vi "_FPGA Send Serial.vi"(4 "error in":errorcluster, 5 "Timeout (5000ms)":u32=5000, 6 "Serial Command":T1={"Port Type"=0, "baud rate (9600)"=9600, "data bits (8)"=8, "stop bits (1)"=10, "parity (0:none)"=0, "DoRead"=FALSE, "Command"=""} {"stop bits (1)" items=["1 bit"=10, "1.5 bits"=15, "2 bits"=20]; "parity (0:none)" items=["None", "Odd", "Even", "Mark", "Space"]; "data bits (8)" min=5 max=8 step=1; "Port Type" items=["RS485", "RS232-1", "RS232-2"]}) -> (0 "error out":errorcluster, 2 "Reply":string)   [LabVIEW 2015]
uses:
  Type/_RT Serial Command.ctl
  Type/_RW Status.ctl
  Type/_FPGA Indicator.ctl
  _RT Global.vi
  <vilib>/Utility/error.llb/Error Cluster From Error Code.vi
  <vilib>/rvi/errors/niLvFpgaAdjustHostInterfaceError.vi
  <vilib>/rvi/interface/nirviReadWriteControl/nirviReadWriteControl.xnode
  Type/FPGA Typedef.ctl
  FPGA Bitfiles/FPGA9607.lvbitx
  NiFpgaLv.dll
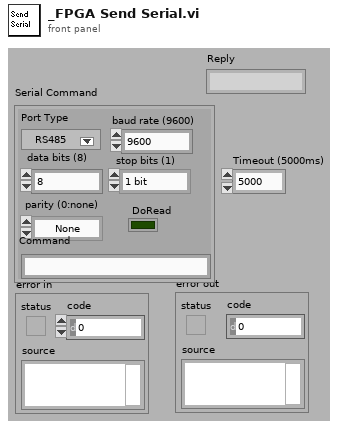
[diagram p1: front panel]
types:
  T1 = typedef "_RT Serial Command.ctl" = cluster{"Port Type":u16, "baud rate (9600)":u32, "data bits (8)":u16, "stop bits (1)":u16, "parity (0:none)":u16, "DoRead":bool, "Command":string}
  T2 = typedef "_RW Status.ctl" = enum8{"Done", "Do Read", "Do Write", "Set Latch1", "Set Latch2", "Set Latch3", "Set Latch4", "RP ON", "EL ON", "Serial Send", "Set LC Out", "Get LC In", "Read VAC", "Table Test", "Get Interlock", "Do Read2", "Do Write2"}
  T3 = typedef "FPGA Typedef.ctl" = refnum<k20>
  T4 = typedef "_FPGA Indicator.ctl" = enum16{"Done", "Ready", "Count Available", "SendSerial", "LED State"}
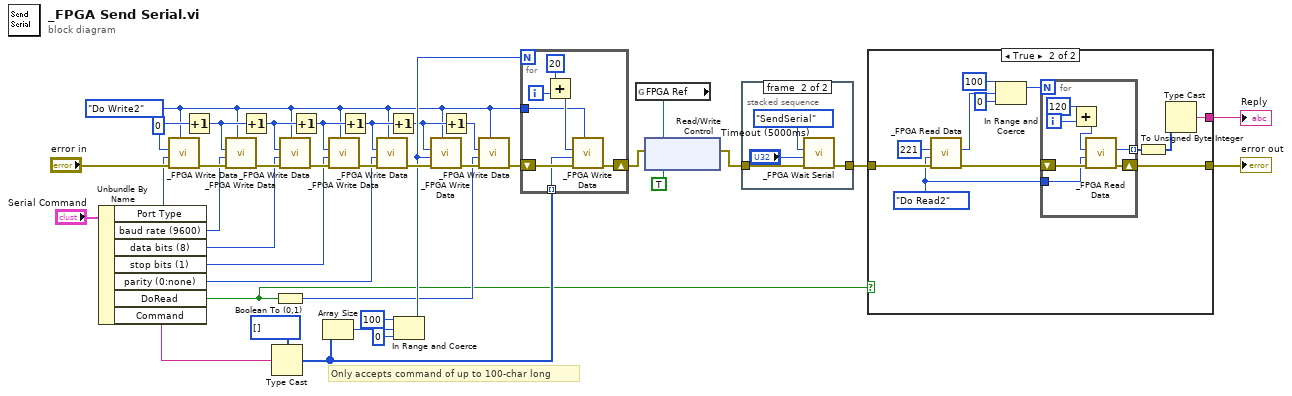
[diagram p0: block diagram]
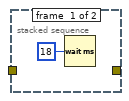
[diagram p3: hidden frame]
diagram:
  w4 = _RW_Status."Do Write2" ("Write Mode (Do Write)")
  w14 = u16 0 ("Address")
  # "Only accepts command of up to 100-char long"
  n1 = Unbundle By Name("Serial Command") -> ("Port Type"=w34:u16, "baud rate (9600)"=w33:u32, "data bits (8)"=w32:u16, "stop bits (1)"=w29:u16, "parity (0:none)"=w28:u16, "DoRead"=w2:bool, "Command"=w15:string)
  n2 = call "_FPGA Write Data.vi"("Write Mode (Do Write)"=w4, "error in"="error in", "Data"=w34, "Address"=w14) -> ("error out"=w37:errorcluster)  [unwired: 2 in, 2 out]
  n3 = Increment(x=w14) -> (x+1=w13:u16)
  n4 = call "_FPGA Write Data.vi"("Write Mode (Do Write)"=w4, "error in"=w37, "Data"=w33, "Address"=w13) -> ("error out"=w36:errorcluster)  [unwired: 2 in, 2 out]
  n5 = Increment(x=w13) -> (x+1=w12:u16)
  n6 = Type Cast(type=u8[] [], x=w15) -> (*(type *) &x=w21:u8[])
  n7 = Boolean To (0,1)(Boolean=w2) -> (0, 1=w8:i16)
  n8 = call "_FPGA Write Data.vi"("Write Mode (Do Write)"=w4, "error in"=w36, "Data"=w32, "Address"=w12) -> ("error out"=w30:errorcluster)  [unwired: 2 in, 2 out]
  n9 = Increment(x=w12) -> (x+1=w11:u16)
  n10 = Array Size(array=w21) -> (size(s)=w25:i32)
  n11 = call "_FPGA Write Data.vi"("Write Mode (Do Write)"=w4, "error in"=w30, "Data"=w29, "Address"=w11) -> ("error out"=w31:errorcluster)  [unwired: 2 in, 2 out]
  n12 = Increment(x=w11) -> (x+1=w10:u16)
  n13 = call "_FPGA Write Data.vi"("Write Mode (Do Write)"=w4, "error in"=w31, "Data"=w28, "Address"=w10) -> ("error out"=w26:errorcluster)  [unwired: 2 in, 2 out]
  n14 = Increment(x=w10) -> (x+1=w7:u16)
  n15 = In Range and Coerce(upper limit=100, x=w25, lower limit=0) -> (coerced(x)=w22:i32)  [unwired: 1 out]
  n16 = call "_FPGA Write Data.vi"("Write Mode (Do Write)"=w4, "error in"=w26, "Data"=w22, "Address"=w7) -> ("error out"=w9:errorcluster)  [unwired: 2 in, 2 out]
  n17 = Increment(x=w7) -> (x+1=w6:u16)
  n18 = call "_FPGA Write Data.vi"("Write Mode (Do Write)"=w4, "error in"=w9, "Data"=w8, "Address"=w6) -> ("error out"=w5:errorcluster)  [unwired: 2 in, 2 out]
  n19 = for {
    N: w22 -> [_]
    shift-right: [w42] -> w3
    shift-left: w5 -> [w43]
    tunnel: w21 -> [w40] mode=indexing
    tunnel: w4 -> [w39]
    i -> [w45]
    n20 = Add(x=20, y=w45) -> (x+y=w41:i32)
    n21 = call "_FPGA Write Data.vi"("Write Mode (Do Write)"=w39, "error in"=w43, "Data"=w40, "Address"=w41) -> ("error out"=w42:errorcluster)  [unwired: 2 in, 2 out]
  }
  n22 = global read "_RT Global.vi" "FPGA Ref"() -> (w1:T3)
  n23 = xnode "Read/Write Control"("FPGA VI Reference In"=w1, "error in"=w3, "Send Serial"=TRUE ("Start")) -> ("error out"=w19:errorcluster)  [unwired: 1 out]
  n24 = stacked-sequence {
    tunnel: w19 -> [_ w49]
    tunnel: [_ w48] -> w18
    frame #0 {
      n25 = Wait (ms)(milliseconds to wait=u32 18) -> ()  [unwired: 1 out]
    }
    frame #1 {
      n26 = call "_FPGA Wait Serial.vi"("error in"=w49, "Timeout (2000ms)"="Timeout (5000ms)", "Indicator"=_FPGA_Indicator."SendSerial") -> ("error out"=w48:errorcluster)  [unwired: 2 in, 2 out]
    }
  }
  n27 = case shown="True" w2 {
    tunnel: w18 -> [w51 w62]
    tunnel: [w51 w60] -> w17
    tunnel: [_ w59] -> w16
    frame False {
    }
    frame True {
      w52 = _RW_Status."Do Read2" ("Read Mode (Do Read)")
      n28 = call "_FPGA Read Data.vi"("error in"=w62, "Read Mode (Do Read)"=w52, "Address"=u16 221) -> ("error out"=w61:errorcluster, "Data"=w55:u32)  [unwired: 2 in, 1 out]
      n29 = In Range and Coerce(upper limit=u32 100, x=w55, lower limit=u32 0) -> (coerced(x)=w56:u32)  [unwired: 1 out]
      n30 = for {
        N: w56 -> [_]
        shift-right: [w67] -> w60
        shift-left: w61 -> [w68]
        tunnel: [w65] -> w58 mode=indexing
        tunnel: w52 -> [w64]
        i -> [w70]
        n31 = Add(x=120, y=w70) -> (x+y=w66:i32)
        n32 = call "_FPGA Read Data.vi"("error in"=w68, "Read Mode (Do Read)"=w64, "Address"=w66) -> ("error out"=w67:errorcluster, "Data"=w65:u32)  [unwired: 1 in, 2 out]
      }
      n33 = To Unsigned Byte Integer(number=w58) -> (unsigned 8bit integer=w57:u8[])
      n34 = Type Cast(x=w57) -> (*(type *) &x=w59:string)  [unwired: 1 out]
    }
  }
  "error out" <- w17
  "Reply" <- w16
